vi "Get Setpoint Notifier.vi"(8 "error in (no error)":errorcluster, 10 "Setpoint Notifier":refnum<notifier>, 11 "PID Loop in":refnum<class "PID Loop.lvclass">) -> (0 "error out":errorcluster, 3 "PID Loop out":refnum<class "PID Loop.lvclass">)   [LabVIEW 2024]
uses:
  PID Loop.lvclass/PID Loop.ctl
  PID Loop.lvclass
  C:/Users/uspoaotto/OneDrive - Oregon Tool/Desktop/working copies/zeroTimeoutMessageHandler/src/Zero Timeout Message Handler/Zero Timeout Message Handler/Zero Timeout Message Handler.lvclass
  C:/Users/uspoaotto/OneDrive - Oregon Tool/Desktop/working copies/zeroTimeoutMessageHandler/samples/PID Controller/PID Loop/PID Loop.lvclass
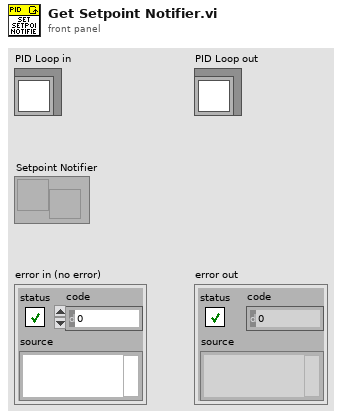
[diagram p1: front panel]
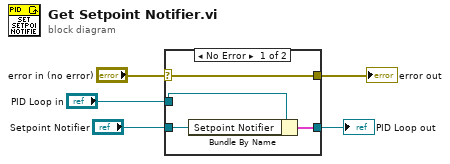
[diagram p0: block diagram]
diagram:
  n1 = case shown="No Error" "error in (no error)" {
    selector: "error in (no error)" -> [w9 w11]
    tunnel: [w9 w11] -> w4
    tunnel: [w7 w10] -> w2
    tunnel: "PID Loop in" -> [w8 w10]
    tunnel: "Setpoint Notifier" -> [w6 _]
    frame No Error {
      n2 = Bundle By Name(cluster=w8, "Setpoint Notifier"=w6) -> (w7:cluster{})
    }
    frame Error {
    }
  }
  "error out" <- w4
  "PID Loop out" <- w2
